vi "Create Reply Sockets.vi"(8 "error in":errorcluster, 9 "Host IP Address":string, 10 "Virt Instrs":T1(array[cluster]), 11 "MSS Target Actor in":refnum<class "MSS Target Actor.lvclass">) -> (0 "error out":errorcluster, 3 "MSS Target Actor out":refnum<class "MSS Target Actor.lvclass">)   [LabVIEW 2023, in "MSS Target Actor.lvlib" / "MSS Target Actor.lvclass"]
uses:
  MSS Target Actor.lvclass
  MSS Target Actor.lvclass/MSS Target Actor.ctl
  Reply Protocol/Reply Protocol DataSocket/Reply Protocol DataSocket.lvclass
  Reply Protocol/Reply Protocol Base/Reply Protocol Base.lvclass/Reply Protocol Base.ctl
  Reply Protocol/Reply Protocol DataSocket/Reply Protocol DataSocket.lvclass/Reply Protocol DataSocket.ctl
  Reply Protocol Manager/Reply Protocol Manager.lvclass
  Reply Protocol/Reply Protocol Base/Reply Protocol Base.lvclass
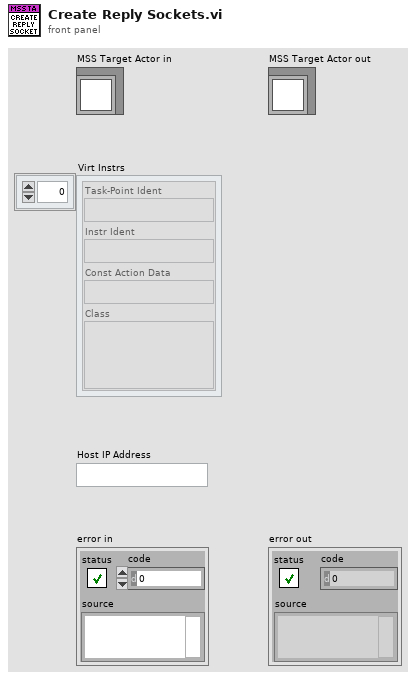
[diagram p1: front panel]
types:
  T1 = cluster{"Task-Point Ident":string, "Instr Ident":string, "Const Action Data":string, "Class":string}[]
  T2 = enum16{"Read", "Write", "ReadWrite", "BufferedRead", "BufferedReadWrite"}
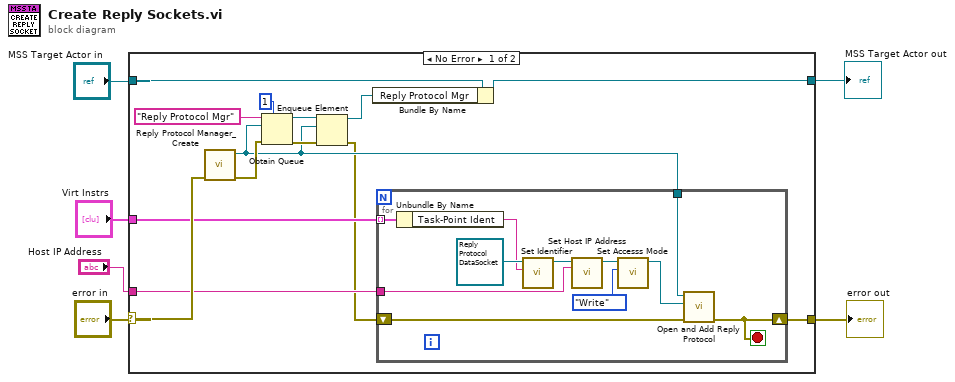
[diagram p0: block diagram]
diagram:
  n1 = case shown="No Error" "error in" {
    selector: "error in" -> [w19 w33]
    tunnel: [w20 w33] -> w4
    tunnel: [w9 w32] -> w3
    tunnel: "MSS Target Actor in" -> [w10 w32]
    tunnel: "Virt Instrs" -> [w18 _]
    tunnel: "Host IP Address" -> [w17 _]
    frame No Error {
      n2 = call "Reply Protocol Manager_Create.vi"("Error In"=w19) -> ("Error Out"=w14:errorcluster, "reference out"=w11:refnum<class "Reply Protocol Manager.lvclass">)  [unwired: 9 in]
      n3 = Obtain Queue(max queue size (-1, unlimited)=1, name (unnamed)="Reply Protocol Mgr", element data type=w11, error in (no error)=w14) -> (queue out=w13:refnum<queue>, error out=w12:errorcluster)  [unwired: 1 in, 1 out]
      n4 = Enqueue Element(queue=w13, element=w11, error in (no error)=w12) -> (queue out=w8:refnum<queue>, error out=w7:errorcluster)  [unwired: 1 in, 1 out]
      n5 = Bundle By Name(cluster=w10, "Reply Protocol Mgr"=w8) -> (w9:refnum<class "MSS Target Actor.lvclass">)
      n6 = for {
        tunnel: w18 -> [w26] mode=indexing
        tunnel: w11 -> [w30]
        shift-right: [w29] -> w20
        shift-left: w7 -> [w31]
        tunnel: w17 -> [w23]
        stop <- w29 stop-if-true
        n7 = Unbundle By Name(w26) -> ("Task-Point Ident"=w25:string)
        n8 = call "Set Identifier.vi"("Identifier"=w25, "Reply Protocol Base in"=refnum<class "Reply Protocol DataSocket.lvclass"> refnum ("HAL GOOP4.lvlib:Reply Protocol DataSocket.lvclass")) -> ("Reply Protocol Base out"=w28:refnum<class "Reply Protocol DataSocket.lvclass">)  [unwired: 9 in]
        n9 = call "Set Host IP Address.vi"("Host IP Address"=w23, "Reply Protocol DataSocket in"=w28) -> ("Reply Protocol DataSocket out"=w24:refnum<class "Reply Protocol DataSocket.lvclass">)  [unwired: 9 in]
        n10 = call "Set Accesss Mode.vi"("Accesss Mode"=T2."Write", "Reply Protocol DataSocket in"=w24) -> ("Reply Protocol DataSocket out"=w22:refnum<class "Reply Protocol DataSocket.lvclass">)  [unwired: 9 in]
        n11 = call "Open and Add Reply Protocol.vi"("Error In"=w31, "Reply Protocol Base"=w22, "reference in"=w30) -> ("Error Out"=w29:errorcluster)  [unwired: 7 in, 1 out]
      }
    }
    frame Error {
    }
  }
  "error out" <- w4
  "MSS Target Actor out" <- w3
